vi "Run Waterfall.vi"(9 "Channel Name":string, 10 "Signal":waveform(dbl)={"t0"=timestamp(0 s since 1904-01-01), "dt"=0.0, "Y"=[]}, 11 "Data":T1={"First Time"=FALSE, "Show Waterfall Button Clicked"=FALSE, "Data to Process"=0.0, "Slice"=0.0, "window"=1, "averaging parameters"={"averaging mode"=enum."No averaging", "weighting mode"=enum."Exponential", "number of averages"=10}, "Waterfall VI Ref"=refnum, "Signal"={"t0"=timestamp(0 s since 1904-01-01), "dt"=0.0, "Y"=[]}} {"averaging parameters"."number of averages" min=1; "window" items=["Rectangle"=0, "Hanning"=1, "Hamming"=2, "Blackman-Harris"=3, "Exact Blackman"=4, "Blackman"=5, "Flat Top"=6, "4 Term B-Harris "=7, "7 Term B-Harris"=8, "Low Sidelobe"=9, "Blackman Nuttall"=11, "Triangle"=30, "Bartlett-Hanning"=31, "Bohman"=32, "Parzen"=33, "Welch"=34, "Kaiser"=60, "Dolph-Chebyshev"=61, "Gaussian"=62]}) -> (3 "Data dup":T1={"First Time"=FALSE, "Show Waterfall Button Clicked"=FALSE, "Data to Process"=0.0, "Slice"=0.0, "window"=1, "averaging parameters"={"averaging mode"=enum."No averaging", "weighting mode"=enum."Exponential", "number of averages"=10}, "Waterfall VI Ref"=refnum, "Signal"={"t0"=timestamp(0 s since 1904-01-01), "dt"=0.0, "Y"=[]}} {"averaging parameters"."number of averages" min=1; "window" items=["Rectangle"=0, "Hanning"=1, "Hamming"=2, "Blackman-Harris"=3, "Exact Blackman"=4, "Blackman"=5, "Flat Top"=6, "4 Term B-Harris "=7, "7 Term B-Harris"=8, "Low Sidelobe"=9, "Blackman Nuttall"=11, "Triangle"=30, "Bartlett-Hanning"=31, "Bohman"=32, "Parzen"=33, "Welch"=34, "Kaiser"=60, "Dolph-Chebyshev"=61, "Gaussian"=62]})   [LabVIEW 2024, in "Waterfall.lvlib" / "Waterfall.lvclass"]
uses:
  Waterfall.lvclass
  Waterfall Data.ctl
  <vilib>/Analysis/4window.llb/windowTd.ctl
  Waterfall.lvclass/Waterfall.ctl
  <vilib>/Analysis/NI_AALPro.lvlib
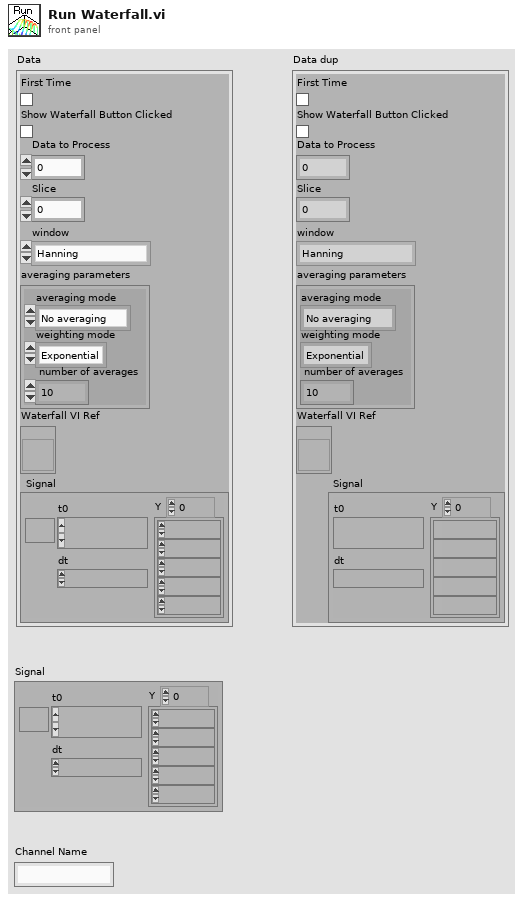
[diagram p1: front panel]
types:
  T1 = typedef "Waterfall.lvlib/Waterfall.lvclass/Waterfall Data.ctl" = cluster{"First Time":bool, "Show Waterfall Button Clicked":bool, "Data to Process":dbl, "Slice":dbl, "window":T2, "averaging parameters":cluster{"averaging mode":enum16{"No averaging", "Vector averaging", "RMS averaging", "Peak hold"}, "weighting mode":enum16{"Linear", "Exponential"}, "number of averages":u32}, "Waterfall VI Ref":refnum<vi>, "Signal":waveform(dbl)}
  T2 = typedef "NI_AALPro.lvlib/windowTd.ctl" = u32
  T3 = cluster{"averaging mode":enum16{"No averaging", "Vector averaging", "RMS averaging", "Peak hold"}, "weighting mode":enum16{"Linear", "Exponential"}, "number of averages":u32}
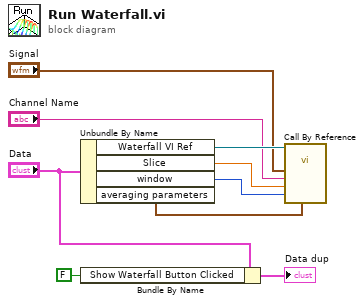
[diagram p0: block diagram]
diagram:
  n1 = Unbundle By Name("Data") -> ("Waterfall VI Ref"=w9:refnum<vi>, "Slice"=w7:dbl, "window"=w6:T2, "averaging parameters"=w4:T3)
  n2 = Bundle By Name(cluster="Data", "Show Waterfall Button Clicked"=FALSE ("First Time")) -> (→"Data dup":T1)
  n3 = call-by-ref "?"(reference=w9, "averaging parameters"=w4, "window"=w6, "Slice"=w7, "Channel Name in"="Channel Name", "Signal"="Signal") -> ()  [unwired: 8 in, 2 out]
